vi "Execute.vi"(8 "error in (no error)":errorcluster, 9 "System in":refnum<class "System.lvclass">, 10 "Command in":refnum<class "Command.lvclass">, 11 "CT-De-Energizing-State in":refnum<class "CT-De-Energizing-State.lvclass">) -> (0 "error out":errorcluster, 2 "Next State":refnum<class "State.lvclass">, 3 "CT-De-Energizing-State out":refnum<class "CT-De-Energizing-State.lvclass">)   [LabVIEW 2013, in "CT-De-Energizing-State.lvclass"]
uses:
  CT-De-Energizing-State.lvclass
  Commands/Command/Command.lvclass
  Systems/System/System.lvclass
  State/State.lvclass
  Systems/Catapult/Catapult.lvclass
  CT-De-Energized-State/CT-De-Energized-State.lvclass
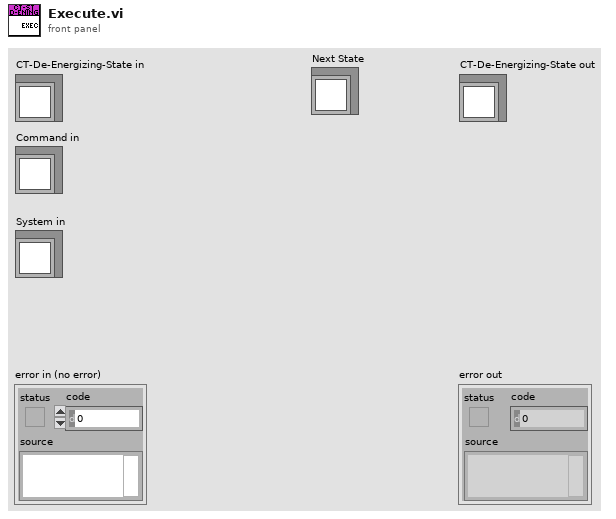
[diagram p1: front panel]
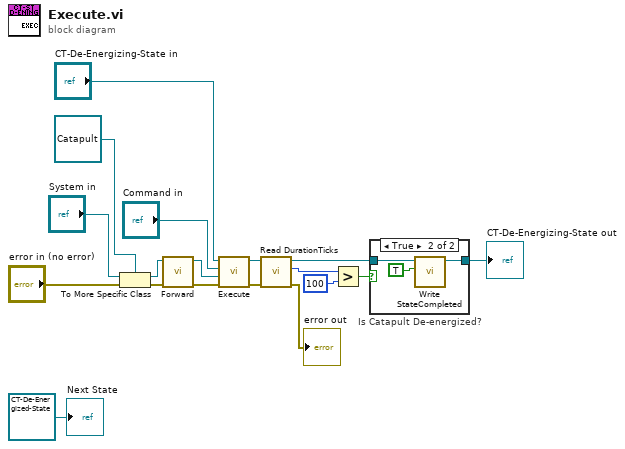
[diagram p0: block diagram]
diagram:
  n1 = To More Specific Class(target class=refnum<class "Catapult.lvclass"> refnum ("Catapult.lvclass"), reference="System in", error in="error in (no error)") -> (specific class reference=w12:refnum<class "Catapult.lvclass">, error out=w10:errorcluster)
  n2 = call-dynamic "Forward.vi"("error in (no error)"=w10, "Catapult in"=w12) -> ("error out"=w9:errorcluster, "Catapult out"=w11:refnum<class "Catapult.lvclass">)  [unwired: 8 in]
  n3 = call-parent "Execute.vi"("error in (no error)"=w9, "System in"=w11, "Command in"="Command in", "State in"="CT-De-Energizing-State in") -> ("error out"=w2:errorcluster, "State out"=w18:refnum<class "CT-De-Energizing-State.lvclass">)  [unwired: 5 in, 1 out]
  n4 = call "Read DurationTicks.vi"("error in (no error)"=w2, "State in"=w18) -> ("error out"=→"error out":errorcluster, "DurationTicks"=w5:u32, "State out"=w7:refnum<class "CT-De-Energizing-State.lvclass">)  [unwired: 7 in]
  n5 = Greater?(x=w5, y=u32 100) -> (0:w3:bool)
  n6 = case "Is Catapult De-energized?" shown="True" w3 {
    tunnel: w7 -> [w19 w22]
    tunnel: [w19 w21] -> w6
    frame False {
    }
    frame True {
      n7 = call-dynamic "Write StateCompleted.vi"("StateCompleted"=TRUE, "State in"=w22) -> ("State out"=w21:refnum<class "CT-De-Energizing-State.lvclass">)  [unwired: 8 in, 1 out]
    }
  }
  "CT-De-Energizing-State out" <- w6
  "Next State" <- refnum<class "CT-De-Energized-State.lvclass"> refnum ("CT-De-Energized-State.lvclass")
